vi "Config Type.vi"(11 "HTTP Command in":refnum<class "HTTP Command.lvclass">) -> (2 "Command Config Type":refnum<class "Command Config.lvclass">)   [LabVIEW 2020, in "VolatusSeq.lvlib" / "HTTP Command.lvclass"]
uses:
  HTTP Command.lvclass
  HTTP Command.lvclass/HTTP Command.ctl
  VolatusSeqConfig/HTTP Command Config/HTTP Command Config.lvclass
  C:/dev/lv20CE/relink/lv-volatus/VolatusSeqConfig/Command Config/Command Config.lvclass
  C:/dev/lv20CE/relink/lv-volatus/VolatusSeqConfig/HTTP Command Config/HTTP Command Config.lvclass
  VolatusSeqConfig/Command Config/Command Config.lvclass
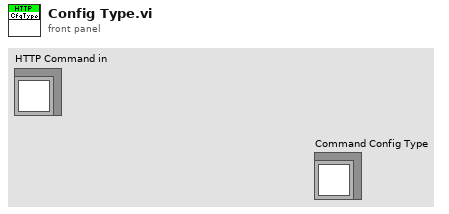
[diagram p1: front panel]
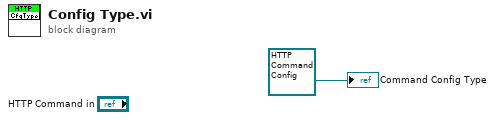
[diagram p0: block diagram]
diagram:
  "Command Config Type" <- refnum<class "HTTP Command Config.lvclass"> refnum ("VolatusSeqConfig.lvlib:HTTP Command Config.lvclass")
